vi "Get Machine ID.vi"(8 "error in (no error)":errorcluster) -> (0 "error out":errorcluster, 2 "machine ID bytes":u8[](array[numeric]) format="%02x", 3 "machine ID":string)   [LabVIEW 2013]
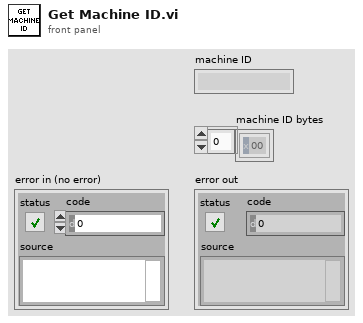
[diagram p1: front panel]
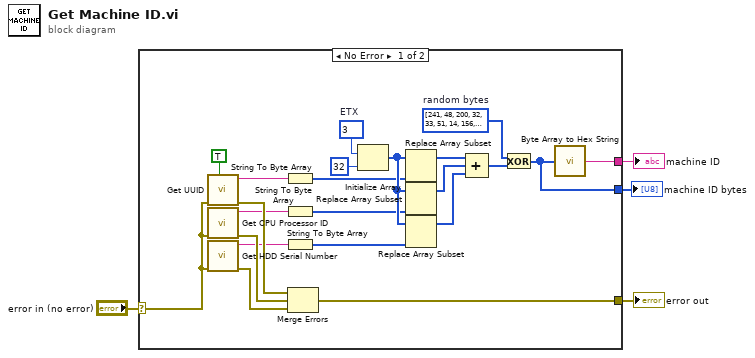
[diagram p0: block diagram]
diagram:
  n1 = case shown="No Error" "error in (no error)" {
    selector: "error in (no error)" -> [w16 w27]
    tunnel: [w21 w27] -> w4
    tunnel: [w13 _] -> w2
    tunnel: [w11 _] -> w1
    frame No Error {
      w10 = u8[] [241, 48, 200, 32, 33, 51, 14, 156, 163, 212, 161, 101, 232, 42, 226, 234, 30, 166, 152, 224, 16, 132, 187, 143, 218, 239, 244, 44, 4, 12, 168, 48]  # random bytes
      w26 = u8 3  # ETX
      n2 = call "Get UUID.vi"("remove hyphen (F)"=TRUE, "error in (no error)"=w16) -> ("error out"=w24:errorcluster, "CSP UUID"=w9:string)  [unwired: 7 in, 1 out]
      n3 = call "Get CPU Processor ID.vi"("error in (no error)"=w16) -> ("error out"=w23:errorcluster, "CPU ID"=w6:string)  [unwired: 8 in, 1 out]
      n4 = call "Get HDD Serial Number.vi"("error in (no error)"=w16) -> ("error out"=w22:errorcluster, "disk drive 0 serial number"=w5:string)  [unwired: 7 in, 2 out]
      n5 = String To Byte Array(string=w9) -> (unsigned byte array=w8:u8[])
      n6 = String To Byte Array(string=w6) -> (unsigned byte array=w7:u8[])
      n7 = String To Byte Array(string=w5) -> (unsigned byte array=w12:u8[])
      n8 = Merge Errors(w24, w23, w22) -> (w21:errorcluster)
      n9 = Initialize Array(w26, 32 ("dimension size")) -> (w25:u8[])
      n10 = Replace Array Subset(array=w25, new element=w8) -> (w19:u8[])  [unwired: 1 in]
      n11 = Replace Array Subset(array=w25, new element=w7) -> (w18:u8[])  [unwired: 1 in]
      n12 = Replace Array Subset(array=w25, new element=w12) -> (w17:u8[])  [unwired: 1 in]
      n13 = Compound Arithmetic op=ADD(w19, w18, w17) -> (w15:u8[])
      n14 = Exclusive Or(1:w15, 2:w10) -> (0:w11:u8[])
      n15 = call "Byte Array to Hex String.vi"("bytes array"=w11) -> ("hex string"=w13:string)
    }
    frame Error {
    }
  }
  "error out" <- w4
  "machine ID" <- w2
  "machine ID bytes" <- w1
